vi "LogisticRegressionCV.vi"(8 "error in":errorcluster) -> (0 "error out":errorcluster, 3 "out":refnum<class "LogisticRegressionCV.lvclass">)   [LabVIEW 2020]
doc: "Logistic Regression CV (aka logit, MaxEnt) classifier.\n\n See glossary entry for :term:`cross-validation estimator`.\n\n This class implements logistic regression using liblinear, newton-cg, sag\n of lbfgs optimizer. The newton-cg, sag and lbfgs solvers support only L2\n regularization with primal formulation. The liblinear solver supports both\n L1 and L2 regularization, with a dual formulation only for the L2 penalty.\n Elastic-Net penalty is only supported by the saga solver.\n\n For the grid of `Cs` values and `l1_ratios` values, the best hyperparameter\n is selected by the cross-validator\n :class:`~sklearn.model_selection.StratifiedKFold`, but it can be changed\n using the :term:`cv` parameter. The 'newton-cg', 'sag', 'saga' and 'lbfgs'\n solvers can warm-start the coefficients (see :term:`Glossary<warm_start>`).\n\n Read more in the :ref:`User Guide <logistic_regression>`.\n\n Parameters\n ----------\n Cs : int or list of floats, default=10\n Each of the values in Cs describes the inverse of regularization\n strength. If Cs is as an int, then a grid of Cs values are chosen\n in a logarithmic scale between 1e-4 and 1e4.\n Like in support vector machines, smaller values specify stronger\n regularization.\n\n fit_intercept : bool, default=True\n Specifies if a constant (a.k.a. bias or intercept) should be\n added to the decision function.\n\n cv : int or cross-validation generator, default=None\n The default cross-validation generator used is Stratified K-Folds.\n If an integer is provided, then it is the number of folds used.\n See the module :mod:`sklearn.model_selection` module for the\n list of possible cross-validation objects.\n\n .. versionchanged:: 0.22\n ``cv`` default value if None changed from 3-fold to 5-fold.\n\n dual : bool, default=False\n Dual or primal formulation. Dual formulation is only implemented for\n l2 penalty with liblinear solver. Prefer dual=False when\n n_samples > n_features.\n\n penalty : {'l1', 'l2', 'elasticnet'}, default='l2'\n Used to specify the norm used in the penalization. The 'newton-cg',\n 'sag' and 'lbfgs' solvers support only l2 penalties. 'elasticnet' is\n only supported by the 'saga' solver.\n\n scoring : str or callable, default=None\n A string (see model evaluation documentation) or\n a scorer callable object / function with signature\n ``scorer(estimator, X, y)``. For a list of scoring functions\n that can be used, look at :mod:`sklearn.metrics`. The\n default scoring option used is 'accuracy'.\n\n solver : {'newton-cg', 'lbfgs', 'liblinear', 'sag', 'saga'}, default='lbfgs'\n\n Algorithm to use in the optimization problem.\n\n - For small datasets, 'liblinear' is a good choice, whereas 'sag' and\n 'saga' are faster for large ones.\n - For multiclass problems, only 'newton-cg', 'sag', 'saga' and 'lbfgs'\n handle multinomial loss; 'liblinear' is limited to one-versus-rest\n schemes.\n - 'newton-cg', 'lbfgs' and 'sag' only handle L2 penalty, whereas\n 'liblinear' and 'saga' handle L1 penalty.\n - 'liblinear' might be slower in LogisticRegressionCV because it does\n not handle warm-starting.\n\n Note that 'sag' and 'saga' fast convergence is only guaranteed on\n features with approximately the same scale. You can preprocess the data\n with a scaler from sklearn.preprocessing.\n\n .. versionadded:: 0.17\n Stochastic Average Gradient descent solver.\n .. versionadded:: 0.19\n SAGA solver.\n\n tol : float, default=1e-4\n Tolerance for stopping criteria.\n\n max_iter : int, default=100\n Maximum number of iterations of the optimization algorithm.\n\n class_weight : dict or 'balanced', default=None\n Weights associated with classes in the form ``{class_label: weight}``.\n If not given, all classes are supposed to have weight one.\n\n The \"balanced\" mode uses the values of y to automatically adjust\n weights inversely proportional to class frequencies in the input data\n as ``n_samples / (n_classes * np.bincount(y))``.\n\n Note that these weights will be multiplied with sample_weight (passed\n through the fit method) if sample_weight is specified.\n\n .. versionadded:: 0.17\n class_weight == 'balanced'\n\n n_jobs : int, default=None\n Number of CPU cores used during the cross-validation loop.\n ``None`` means 1 unless in a :obj:`joblib.parallel_backend` context.\n ``-1`` means using all processors. See :term:`Glossary <n_jobs>`\n for more details.\n\n verbose : int, default=0\n For the 'liblinear', 'sag' and 'lbfgs' solvers set verbose to any\n positive number for verbosity.\n\n refit : bool, default=True\n If set to True, the scores are averaged across all folds, and the\n coefs and the C that corresponds to the best score is taken, and a\n final refit is done using these parameters.\n Otherwise the coefs, intercepts and C that correspond to the\n best scores across folds are averaged.\n\n intercept_scaling : float, default=1\n Useful only when the solver 'liblinear' is used\n and self.fit_intercept is set to True. In this case, x becomes\n [x, self.intercept_scaling],\n i.e. a \"synthetic\" feature with constant value equal to\n intercept_scaling is appended to the instance vector.\n The intercept becomes ``intercept_scaling * synthetic_feature_weight``.\n\n Note! the synthetic feature weight is subject to l1/l2 regularization\n as all other features.\n To lessen the effect of regularization on synthetic feature weight\n (and therefore on the intercept) intercept_scaling has to be increased.\n\n multi_class : {'auto, 'ovr', 'multinomial'}, default='auto'\n If the option chosen is 'ovr', then a binary problem is fit for each\n label. For 'multinomial' the loss minimised is the multinomial loss fit\n across the entire probability distribution, *even when the data is\n binary*. 'multinomial' is unavailable when solver='liblinear'.\n 'auto' selects 'ovr' if the data is binary, or if solver='liblinear',\n and otherwise selects 'multinomial'.\n\n .. versionadded:: 0.18\n Stochastic Average Gradient descent solver for 'multinomial' case.\n .. versionchanged:: 0.22\n Default changed from 'ovr' to 'auto' in 0.22.\n\n random_state : int, RandomState instance, default=None\n Used when `solver='sag'`, 'saga' or 'liblinear' to shuffle the data.\n Note that this only applies to the solver and not the cross-validation\n generator. See :term:`Glossary <random_state>` for details.\n\n l1_ratios : list of float, default=None\n The list of Elastic-Net mixing parameter, with ``0 <= l1_ratio <= 1``.\n Only used if ``penalty='elasticnet'``. A value of 0 is equivalent to\n using ``penalty='l2'``, while 1 is equivalent to using\n ``penalty='l1'``. For ``0 < l1_ratio <1``, the penalty is a combination\n of L1 and L2.\n\n Attributes\n ----------\n classes_ : ndarray of shape (n_classes, )\n A list of class labels known to the classifier.\n\n coef_ : ndarray of shape (1, n_features) or (n_classes, n_features)\n Coefficient of the features in the decision function.\n\n `coef_` is of shape (1, n_features) when the given problem\n is binary.\n\n intercept_ : ndarray of shape (1,) or (n_classes,)\n Intercept (a.k.a. bias) added to the decision function.\n\n If `fit_intercept` is set to False, the intercept is set to zero.\n `intercept_` is of shape(1,) when the problem is binary.\n\n Cs_ : ndarray of shape (n_cs)\n Array of C i.e. inverse of regularization parameter values used\n for cross-validation.\n\n l1_ratios_ : ndarray of shape (n_l1_ratios)\n Array of l1_ratios used for cross-validation. If no l1_ratio is used\n (i.e. penalty is not 'elasticnet'), this is set to ``[None]``\n\n coefs_paths_ : ndarray of shape (n_folds, n_cs, n_features) or (n_folds, n_cs, n_features + 1)\n dict with classes as the keys, and the path of coefficients obtained\n during cross-validating across each fold and then across each Cs\n after doing an OvR for the corresponding class as values.\n If the 'multi_class' option is set to 'multinomial', then\n the coefs_paths are the coefficients corresponding to each class.\n Each dict value has shape ``(n_folds, n_cs, n_features)`` or\n ``(n_folds, n_cs, n_features + 1)`` depending on whether the\n intercept is fit or not. If ``penalty='elasticnet'``, the shape is\n ``(n_folds, n_cs, n_l1_ratios_, n_features)`` or\n ``(n_folds, n_cs, n_l1_ratios_, n_features + 1)``.\n\n scores_ : dict\n dict with classes as the keys, and the values as the\n grid of scores obtained during cross-validating each fold, after doing\n an OvR for the corresponding class. If the 'multi_class' option\n given is 'multinomial' then the same scores are repeated across\n all classes, since this is the multinomial class. Each dict value\n has shape ``(n_folds, n_cs`` or ``(n_folds, n_cs, n_l1_ratios)`` if\n ``penalty='elasticnet'``.\n\n C_ : ndarray of shape (n_classes,) or (n_classes - 1,)\n Array of C that maps to the best scores across every class. If refit is\n set to False, then for each class, the best C is the average of the\n C's that correspond to the best scores for each fold.\n `C_` is of shape(n_classes,) when the problem is binary.\n\n l1_ratio_ : ndarray of shape (n_classes,) or (n_classes - 1,)\n Array of l1_ratio that maps to the best scores across every class. If\n refit is set to False, then for each class, the best l1_ratio is the\n average of the l1_ratio's that correspond to the best scores for each\n fold. `l1_ratio_` is of shape(n_classes,) when the problem is binary.\n\n n_iter_ : ndarray of shape (n_classes, n_folds, n_cs) or (1, n_folds, n_cs)\n Actual number of iterations for all classes, folds and Cs.\n In the binary or multinomial cases, the first dimension is equal to 1.\n If ``penalty='elasticnet'``, the shape is ``(n_classes, n_folds,\n n_cs, n_l1_ratios)`` or ``(1, n_folds, n_cs, n_l1_ratios)``.\n\n\n \nAvailable methods:\nGet Attributes\nGet Params\nSet Params"
uses:
  LogisticRegressionCV.lvclass
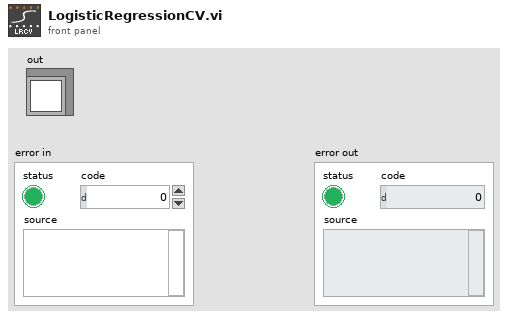
[diagram p1: front panel]
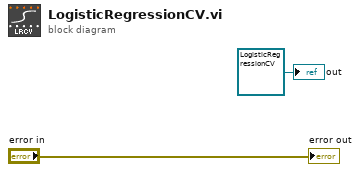
[diagram p0: block diagram]
diagram:
  "out" <- refnum<class "LogisticRegressionCV.lvclass"> refnum ("model")
  "error out" <- "error in"
